vi "DataToRead.vi"(8 "error in (no error)":errorcluster, 11 "MultiReader in":refnum<class "MultiReader.lvclass">) -> (0 "error out":errorcluster, 2 "Data available?":bool, 3 "MultiReader out":refnum<class "MultiReader.lvclass">)   [LabVIEW 2025, in "MultiReader.lvclass"]
doc: "Returns TRUE if there is any data to read from the remote host"
uses:
  MultiReader.lvclass
  MultiReader.lvclass/MultiReader.ctl
  BaseReader/BaseReader.lvclass
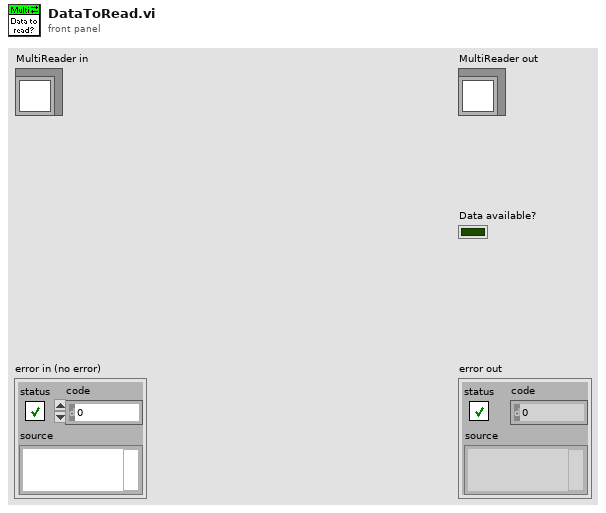
[diagram p1: front panel]
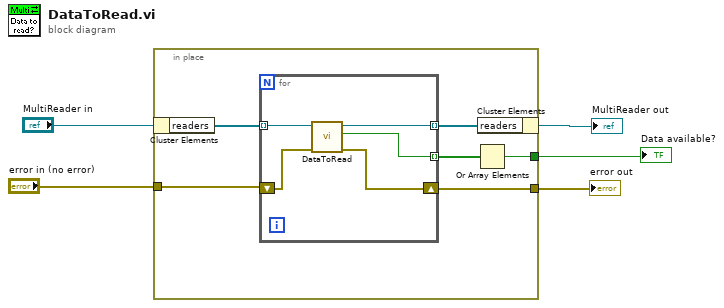
[diagram p0: block diagram]
diagram:
  n1 = in-place {
    in-place-border: "error in (no error)" -> [w9]
    in-place-border: [w8] -> w3
    in-place-border: [w6] -> w1
    n2 = in-place-cluster #1("MultiReader in") -> ("readers"=w11:refnum<class "BaseReader.lvclass">[])
    n3 = for {
      tunnel: w11 -> [w16] mode=indexing
      tunnel: [w15] -> w10 mode=indexing
      tunnel: [w14] -> w7 mode=indexing
      shift-right: [w13] -> w8
      shift-left: w9 -> [w12]
      n4 = call-dynamic "DataToRead.vi"("error in (no error)"=w12, "BaseReader in"=w16) -> ("error out"=w13:errorcluster, "Data available?"=w14:bool, "BaseReader out"=w15:refnum<class "BaseReader.lvclass">)  [unwired: 7 in]
    }
    n5 = Or Array Elements(Boolean array=w7) -> (logical OR=w6:bool)
    n6 = in-place-cluster #1("readers"=w10) -> (→"MultiReader out":refnum<class "MultiReader.lvclass">)
  }
  "error out" <- w3
  "Data available?" <- w1
